vi "updateStorage.vi"(8 "error in (no error)":errorcluster, 9 "IN-OUT":bool, 10 "dataIN":string[][](array[string]), 11 "reference in":refnum<class "Items Controller.lvclass">) -> (0 "error out":errorcluster, 2 "warningMess":string[](array[string]), 3 "reference out":refnum<class "Items Controller.lvclass">)   [LabVIEW 2014, in "Items Controller.lvclass"]
uses:
  Items Controller.lvclass
  IN-OUT-state.ctl
  APP/item_class/item.lvclass
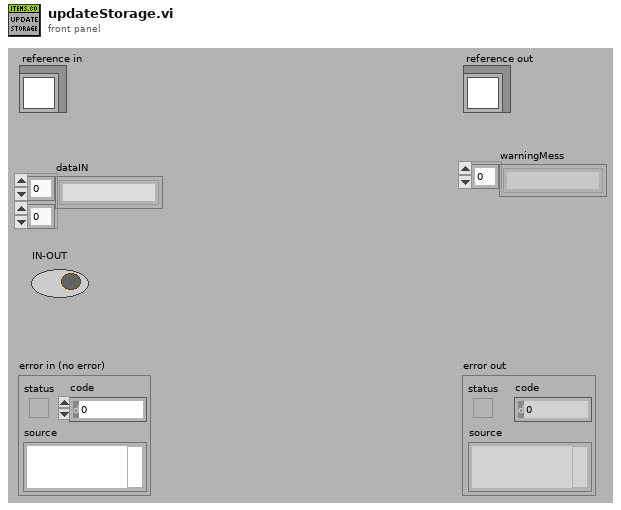
[diagram p1: front panel]
types:
  T1 = typedef "Items Controller.lvclass/IN-OUT-state.ctl" = enum16{"firstCheck", "onlyQnt", "nextItem", "secondCheck", "checkState", "addItems", "updateItems", "numS/N", "stop"}
  T2 = typedef "Items Controller.lvclass/ObjectAttributesRef.ctl" = refnum<data-value>
  T3 = typedef "Items Controller.lvclass/ObjectAttributes.ctl" = cluster{"MyAttribute":dbl, "data":string[][][], "file_controller_ref":refnum<class "File Controller.lvclass">, "checkIN_ref":refnum<class "checkIN.lvclass">, "checkOUT_ref":refnum<class "checkOUT.lvclass">, "item_ref":refnum<class "item.lvclass">}
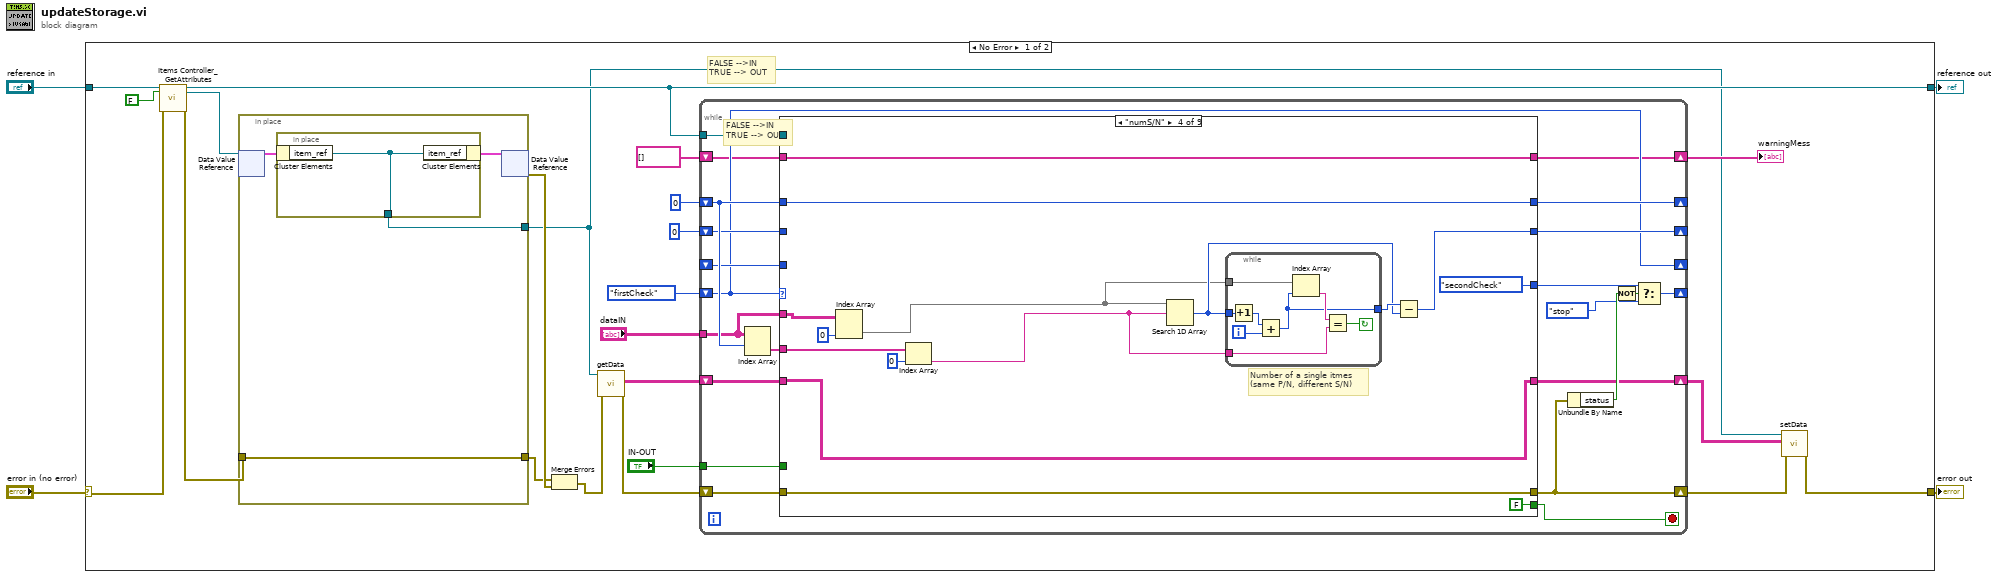
[diagram p0: block diagram]
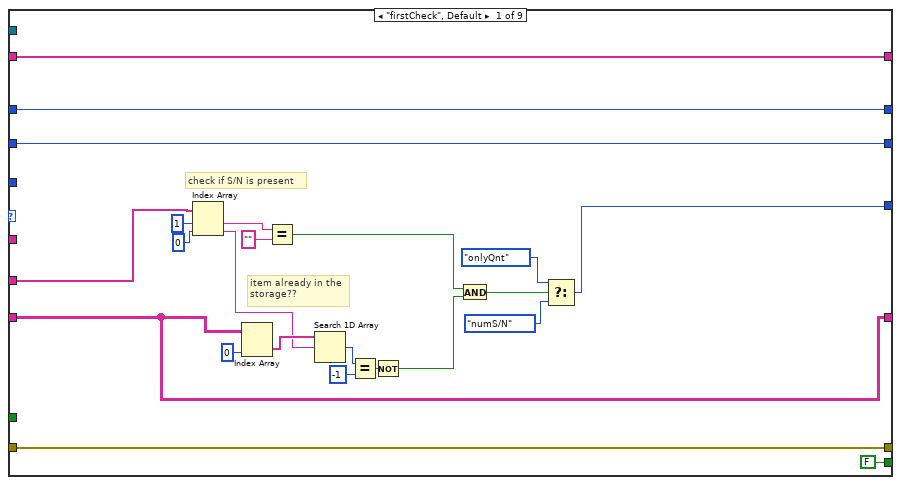
[diagram p2: hidden frame]
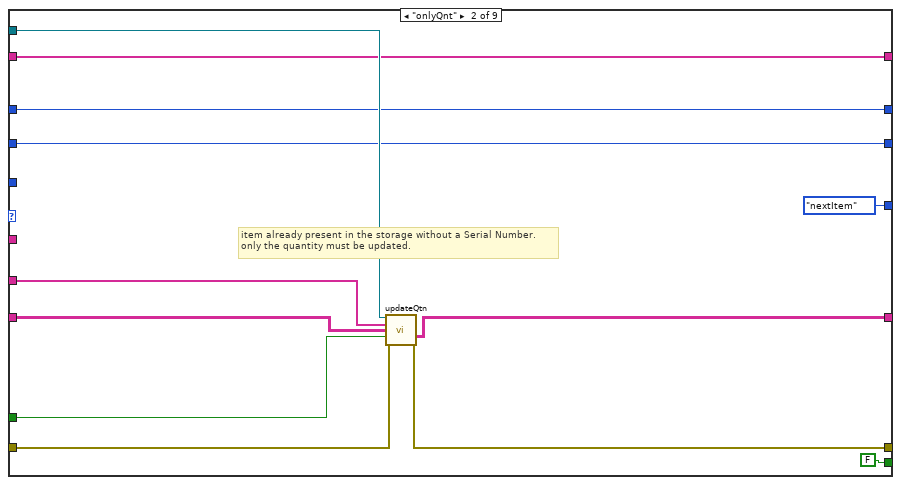
[diagram p3: hidden frame]
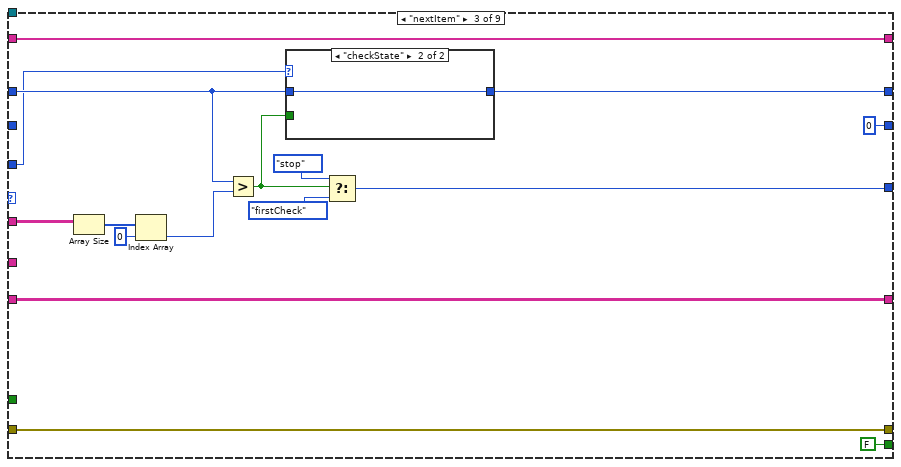
[diagram p4: hidden frame]
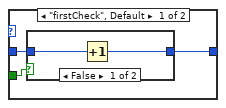
[diagram p5: hidden frame]
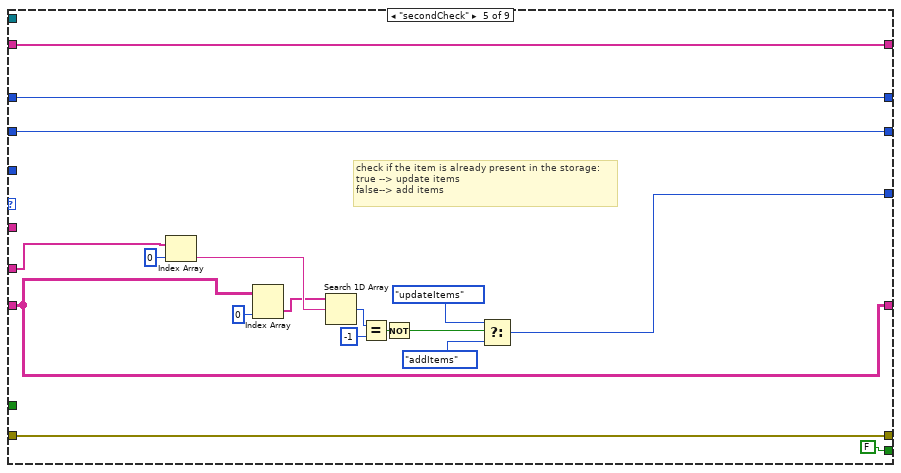
[diagram p7: hidden frame]
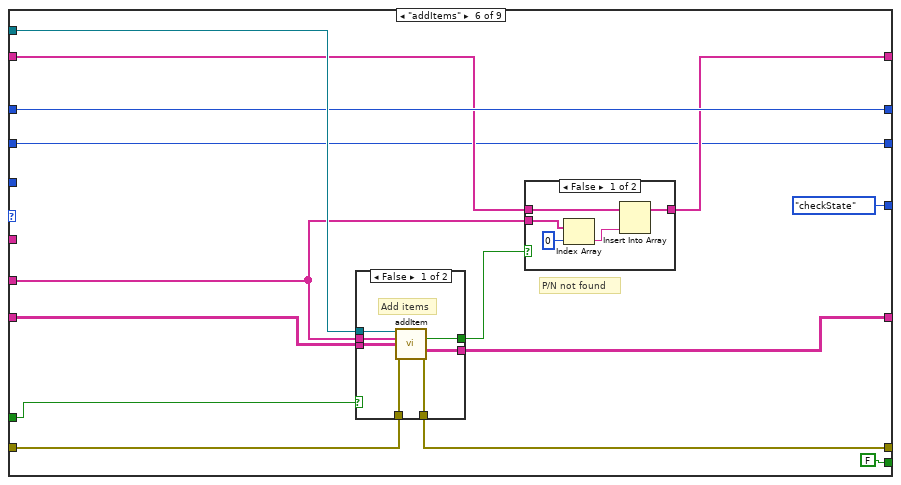
[diagram p8: hidden frame]
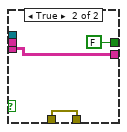
[diagram p9: hidden frame]
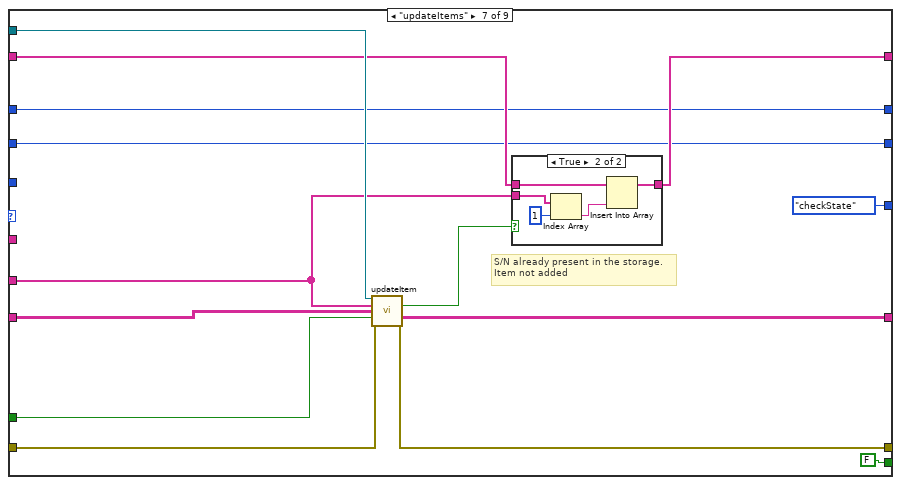
[diagram p11: hidden frame]
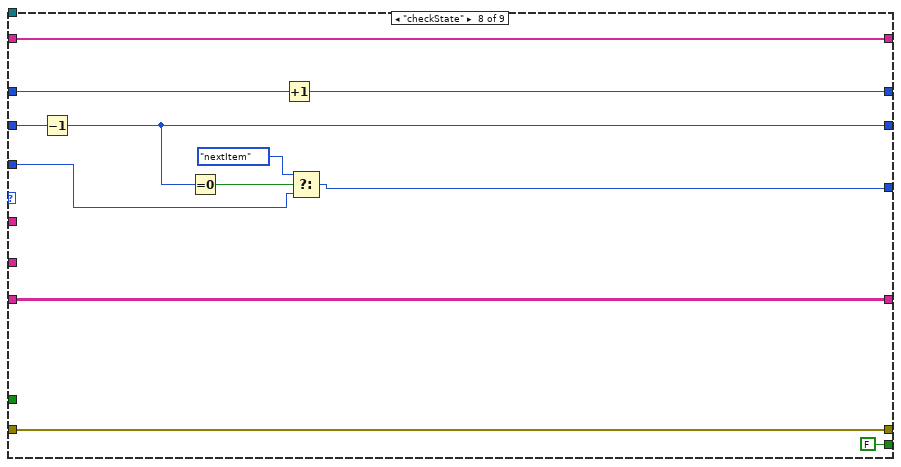
[diagram p13: hidden frame]
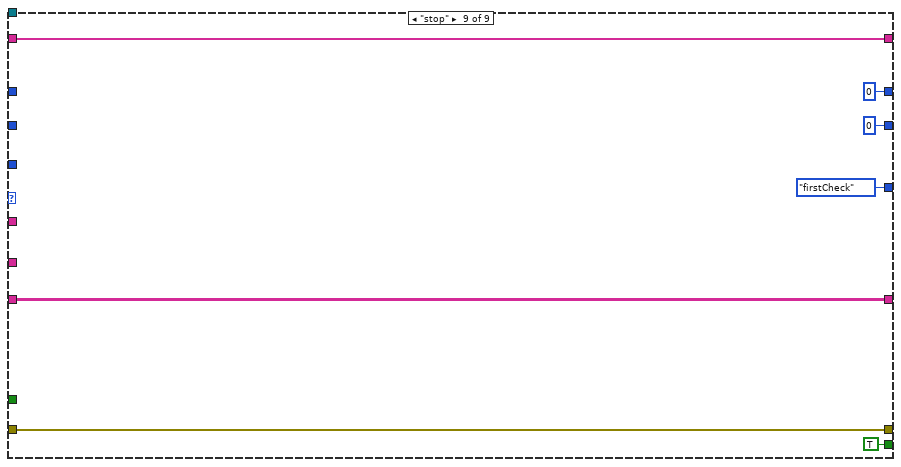
[diagram p14: hidden frame]
diagram:
  n1 = case shown="No Error" "error in (no error)" {
    selector: "error in (no error)" -> [w22 w223]
    tunnel: [w5 w223] -> w3
    tunnel: [w13 w222] -> w1
    tunnel: "reference in" -> [w24 w222]
    frame No Error {
      # "FALSE -->IN\nTRUE --> OUT"
      # "FALSE -->IN\nTRUE --> OUT"
      n2 = call "Items Controller_GetAttributes.vi"("reference in"=w24, "return data? (T)"=FALSE, "error in (no error)"=w22) -> ("reference out"=w13:refnum<class "Items Controller.lvclass">, "attributes ref"=w20:T2, "error out"=w21:errorcluster)  [unwired: 13 in, 1 out]
      n3 = in-place {
        in-place-border: w21 -> [w218]
        in-place-border: [w218] -> w25
        in-place-border: [w217] -> w8
        n4 = in-place-dvr #1(w20) -> (w219:T3)  [unwired: 1 out]
        n5 = in-place {
          in-place-border: [w221] -> w217
          n6 = in-place-cluster #2(w219) -> ("item_ref"=w221:refnum<class "item.lvclass">)
          n7 = in-place-cluster #2("item_ref"=w221) -> (w220:T3)
        }
        n8 = in-place-dvr #1(w220) -> (w26:errorcluster)  [unwired: 1 out]
      }
      n9 = Merge Errors(w25, w26) -> (w19:errorcluster)
      n10 = call "getData.vi"("error in (no error)"=w19, "reference in"=w8) -> ("error out"=w17:errorcluster, "data"=w15:string[][])  [unwired: 7 in, 1 out]
      n11 = while {
        shift-right: [w39] -> _
        shift-left: IN-OUT-state."firstCheck" ("state") -> [w30]
        shift-right: [w46] -> w6
        shift-left: w17 -> [w47]
        tunnel: "dataIN" -> [w35]
        shift-right: [w40] -> w7
        shift-left: w15 -> [w43]
        tunnel: "IN-OUT" -> [w42]
        tunnel: w13 -> [w41]
        shift-right: [w38] -> _
        shift-left: 0 -> [w37]
        shift-right: [w33] -> _
        shift-left: 0 -> [w34]
        shift-right: [w30] -> _
        shift-left: _ -> [w31]
        shift-right: [w28] -> w9
        shift-left: string[] [] -> [w29]
        stop <- w48 stop-if-true
        n12 = Index Array(array=w35, index (row)=w37) -> (element=w36:string[])  [unwired: 1 in]
        n13 = case shown="\"numS/N\"" w30 {
          tunnel: [FALSE FALSE FALSE FALSE FALSE FALSE FALSE FALSE TRUE] -> w48
          tunnel: w47 -> [w70 w81 w99 w117 w146 w160 w188 w207 w215]
          tunnel: [w70 w80 w99 w117 w146 w159 w187 w207 w215] -> w46
          tunnel: w36 -> [w52 w75 _ w111 w140 w153 w183 _ _]
          tunnel: w43 -> [w53 w79 w97 w113 w139 w157 w190 w205 w214]
          tunnel: [w54 IN-OUT-state."nextItem" ("state") w90 IN-OUT-state."secondCheck" ("state") w134 IN-OUT-state."checkState" ("state") IN-OUT-state."checkState" ("state") w201 IN-OUT-state."firstCheck" ("state")] -> w32
          tunnel: w42 -> [_ w82 _ _ _ w148 w189 _ _]
          tunnel: w41 -> [_ w78 _ _ _ w158 w186 _ _]
          tunnel: [w53 w77 w97 w113 w139 w156 w185 w205 w214] -> w40
          tunnel: w37 -> [w51 w74 w88 w114 w138 w155 w180 w209 _]
          tunnel: [w51 w74 w87 w114 w138 w155 w180 w200 0] -> w38
          tunnel: w35 -> [_ _ w96 w110 _ _ _ _ _]
          tunnel: w34 -> [w50 w73 _ _ w131 w149 w179 w208 _]
          tunnel: [w50 w73 0 w115 w131 w149 w179 w204 0] -> w33
          tunnel: w31 -> [_ _ w84 _ _ _ _ w202 _]
          tunnel: w29 -> [w49 w72 w86 w112 w130 w152 w182 w198 w210]
          tunnel: [w49 w72 w86 w112 w130 w151 w181 w198 w210] -> w28
          frame "firstCheck", Default {
            # "item already in the\nstorage??"
            # "check if S/N is present"
            n14 = Index Array(array=w52, index #1=1 ("index"), index #2=0 ("index")) -> (element #1=w68:string, element #2=w60:string)
            n15 = Index Array(array=w53, index (col)=0 ("index (row)")) -> (element=w65:string[])  [unwired: 1 in]
            n16 = Equal?(x=w68, y="") -> (x = y?=w58:bool)
            n17 = Search 1D Array(1D array=w65, element=w60) -> (index of element=w64:i32)  [unwired: 1 in]
            n18 = Equal?(x=w64, y=-1) -> (x = y?=w62:bool)
            n19 = Not(x=w62) -> (.not. x?=w59:bool)
            n20 = And(x=w58, y=w59) -> (x .and. y?=w57:bool)
            n21 = Select(t=IN-OUT-state."onlyQnt" ("state"), s=w57, f=IN-OUT-state."numS/N" ("state")) -> (s? t:f=w54:T1)
          }
          frame "onlyQnt" {
            # "item already present in the storage without a Serial Number.\nonly the quantity must be updated."
            n22 = call "updateQtn.vi"("reference in"=w78, "dataIN"=w75, "storageIN"=w79, "IN-OUT"=w82, "error in (no error)"=w81) -> ("storageOUT"=w77:string[][], "error out"=w80:errorcluster)  [unwired: 7 in, 2 out]
          }
          frame "nextItem" {
            n23 = Array Size(array=w96) -> (size(s)=w95:i32[])
            n24 = Index Array(array=w95, index=0) -> (element=w93:i32)
            n25 = Greater?(x=w88, y=w93) -> (0:w89:bool)
            n26 = case shown="\"checkState\"" w84 {
              tunnel: w89 -> [w102 _]
              tunnel: w88 -> [w101 w106]
              tunnel: [w100 w106] -> w87
              frame "firstCheck", Default {
                n27 = case shown="False" w102 {
                  tunnel: w101 -> [w104 w105]
                  tunnel: [w103 w105] -> w100
                  frame False {
                    n28 = Increment(x=w104) -> (x+1=w103:i32)
                  }
                  frame True {
                  }
                }
              }
              frame "checkState" {
              }
            }
            n29 = Select(t=IN-OUT-state."stop" ("state"), s=w89, f=IN-OUT-state."firstCheck" ("state")) -> (s? t:f=w90:T1)
          }
          frame "numS/N" {
            # "Number of a single itmes \n(same P/N, different S/N)"
            n30 = Index Array(array=w110, index (col)=0 ("disabled index (col)")) -> (element=w108:string[])  [unwired: 1 in]
            n31 = Index Array(array=w111, index=0) -> (element=w118:string)
            n32 = Search 1D Array(1D array=w108, element=w118) -> (index of element=w119:i32)  [unwired: 1 in]
            n33 = while {
              tunnel: w108 -> [w129]
              tunnel: w119 -> [w124]
              tunnel: w118 -> [w125]
              tunnel: [w123] -> w120
              i -> [w128]
              stop <- w127 continue-if-true
              n34 = Increment(x=w124) -> (x+1=w122:i32)
              n35 = Add(x=w122, y=w128) -> (x+y=w123:i32)
              n36 = Index Array(array=w129, index=w123) -> (element=w126:string)
              n37 = Equal?(x=w126, y=w125) -> (x = y?=w127:bool)
            }
            n38 = Subtract(x=w120, y=w119) -> (x-y=w115:i32)
          }
          frame "secondCheck" {
            # "check if the item is already present in the storage:\ntrue --> update items\nfalse--> add items"
            n39 = Index Array(array=w140, index=0) -> (element=w133:string)
            n40 = Index Array(array=w139, index (col)=0 ("index (row)")) -> (element=w132:string[])  [unwired: 1 in]
            n41 = Search 1D Array(1D array=w132, element=w133) -> (index of element=w143:i32)  [unwired: 1 in]
            n42 = Equal?(x=w143, y=-1) -> (x = y?=w141:bool)
            n43 = Not(x=w141) -> (.not. x?=w137:bool)
            n44 = Select(t=IN-OUT-state."updateItems" ("state"), s=w137, f=IN-OUT-state."addItems" ("state")) -> (s? t:f=w134:T1)
          }
          frame "addItems" {
            # "P/N not found"
            n45 = case shown="False" w148 {
              tunnel: w160 -> [w168 w171]
              tunnel: [w167 w171] -> w159
              tunnel: w158 -> [w166 _]
              tunnel: w157 -> [w165 w170]
              tunnel: [w164 w170] -> w156
              tunnel: w153 -> [w163 _]
              tunnel: [w162 FALSE ("found?")] -> w150
              frame False {
                # "Add items"
                n46 = call "addItem.vi"("reference in"=w166, "dataIN"=w163, "storageIN"=w165, "error in (no error)"=w168) -> ("found?"=w162:bool, "storageOUT"=w164:string[][], "error out"=w167:errorcluster)  [unwired: 8 in, 1 out]
              }
              frame True {
              }
            }
            n47 = case shown="False" w150 {
              tunnel: w152 -> [w176 w177]
              tunnel: [w175 w177] -> w151
              tunnel: w153 -> [w174 _]
              frame False {
                n48 = Index Array(array=w174, index=0) -> (element=w172:string)
                n49 = Insert Into Array(array=w176, new element=w172) -> (w175:string[])  [unwired: 1 in]
              }
              frame True {
              }
            }
          }
          frame "updateItems" {
            # "S/N already present in the storage.\nItem not added"
            n50 = call "updateItem.vi"("reference in"=w186, "dataIN"=w183, "storageIN"=w190, "IN/OUT"=w189, "error in (no error)"=w188) -> ("found?"=w184:bool, "storageOUT"=w185:string[][], "error out"=w187:errorcluster)  [unwired: 7 in, 1 out]
            n51 = case shown="True" w184 {
              tunnel: w182 -> [w192 w197]
              tunnel: [w192 w196] -> w181
              tunnel: w183 -> [_ w195]
              frame False {
              }
              frame True {
                n52 = Index Array(array=w195, index=1) -> (element=w193:string)
                n53 = Insert Into Array(array=w197, new element=w193) -> (w196:string[])  [unwired: 1 in]
              }
            }
          }
          frame "checkState" {
            n54 = Decrement(x=w208) -> (x-1=w204:i32)
            n55 = Equal To 0?(x=w204) -> (x = 0?=w203:bool)
            n56 = Increment(x=w209) -> (x+1=w200:i32)
            n57 = Select(t=IN-OUT-state."nextItem", s=w203, f=w202) -> (s? t:f=w201:T1)
          }
          frame "stop" {
          }
        }
        n58 = Unbundle By Name(w46) -> ("status"=w45:bool)
        n59 = Not(x=w45) -> (.not. x?=w27:bool)
        n60 = Select(t=w32, s=w27, f=IN-OUT-state."stop" ("state")) -> (s? t:f=w39:T1)
      }
      "warningMess" <- w9
      n61 = call "setData.vi"("error in (no error)"=w6, "data"=w7, "reference in"=w8) -> ("error out"=w5:errorcluster)  [unwired: 7 in, 1 out]
    }
    frame Error {
    }
  }
  "error out" <- w3
  "reference out" <- w1
